vi "MoveOneStep.vi"(8 "error in (no error)":errorcluster, 11 "SnakeBodyUnit in":refnum<class "SnakeBodyCell.lvclass">) -> (0 "error out":errorcluster, 3 "SnakeBodyUnit out":refnum<class "SnakeBodyCell.lvclass">)   [LabVIEW 2018, in "SnakeBodyCell.lvclass"]
uses:
  SnakeBodyCell.lvclass
  SnakeBodyCell.lvclass/SnakeBodyCell.ctl
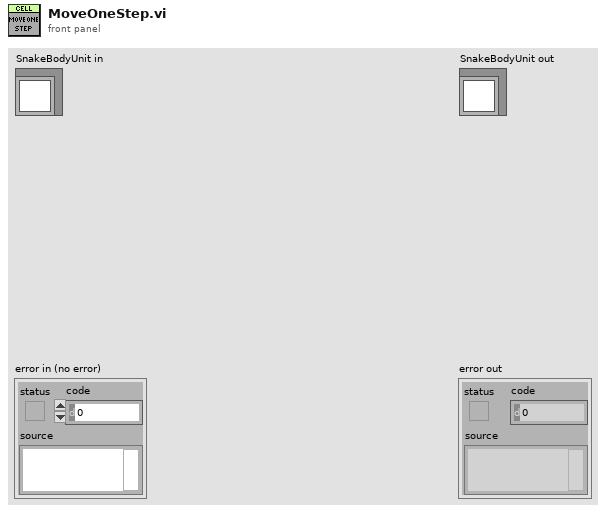
[diagram p1: front panel]
types:
  T1 = typedef "UnitDirection.ctl" = enum16{"North", "East", "South", "West"}
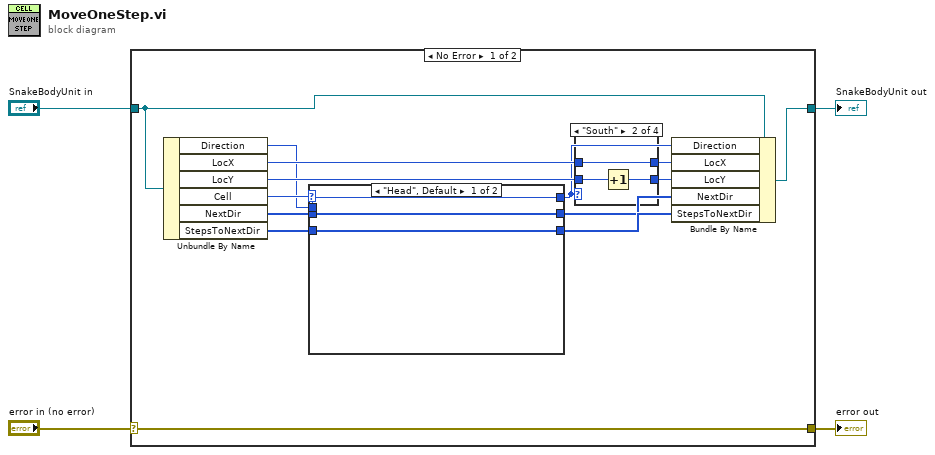
[diagram p0: block diagram]
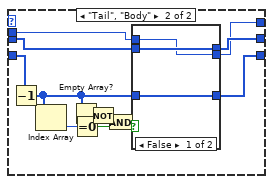
[diagram p2: hidden frame]
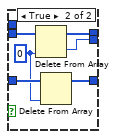
[diagram p3: hidden frame]
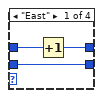
[diagram p4: hidden frame]
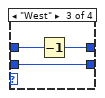
[diagram p5: hidden frame]
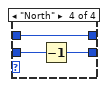
[diagram p6: hidden frame]
diagram:
  n1 = case shown="No Error" "error in (no error)" {
    selector: "error in (no error)" -> [w18 w56]
    tunnel: [w18 w56] -> w3
    tunnel: [w16 w55] -> w1
    tunnel: "SnakeBodyUnit in" -> [w17 w55]
    frame No Error {
      n2 = Unbundle By Name(w17) -> ("Direction"=w7:T1, "LocX"=w14:u16, "LocY"=w12:u16, "Cell"=w11:enum16{"Head", "Tail", "Body"}, "NextDir"=w9:T1[], "StepsToNextDir"=w10:u16[])
      n3 = case shown="\"Head\", Default" w11 {
        tunnel: w10 -> [w20 w33]
        tunnel: w9 -> [w19 w31]
        tunnel: [w20 w29] -> w8
        tunnel: [w21 w28] -> w5
        tunnel: w7 -> [w21 w26]
        tunnel: [w19 w30] -> w6
        frame "Head", Default {
        }
        frame "Tail", "Body" {
          n4 = Decrement(x=w33) -> (x-1=w23:u16[])
          n5 = Index Array(array=w23) -> (element=w32:u16)  [unwired: 1 in]
          n6 = Empty Array?(array=w23) -> (empty?=w24:bool)
          n7 = Equal To 0?(x=w32) -> (x = 0?=w27:bool)
          n8 = Not(x=w24) -> (.not. x?=w22:bool)
          n9 = And(x=w22, y=w27) -> (x .and. y?=w25:bool)
          n10 = case shown="False" w25 {
            tunnel: w23 -> [w35 w42]
            tunnel: w31 -> [w36 w41]
            tunnel: [w36 w40] -> w30
            tunnel: [w35 w39] -> w29
            tunnel: [w34 w37] -> w28
            tunnel: w26 -> [w34 _]
            frame False {
            }
            frame True {
              w38 = 0 ("index")
              n11 = Delete From Array(array=w41, index=w38) -> (deleted portion=w37:T1, array with subset deleted=w40:T1[])  [unwired: 1 in]
              n12 = Delete From Array(array=w42, index=w38) -> (array with subset deleted=w39:u16[])  [unwired: 1 in, 1 out]
            }
          }
        }
      }
      n13 = case shown="\"South\"" w5 {
        tunnel: [w43 w48 w49 w54] -> w15
        tunnel: w14 -> [w45 w48 w51 w54]
        tunnel: [w44 w46 w50 w52] -> w13
        tunnel: w12 -> [w44 w47 w50 w53]
        frame "East" {
          n14 = Increment(x=w45) -> (x+1=w43:u16)
        }
        frame "South" {
          n15 = Increment(x=w47) -> (x+1=w46:u16)
        }
        frame "West" {
          n16 = Decrement(x=w51) -> (x-1=w49:u16)
        }
        frame "North" {
          n17 = Decrement(x=w53) -> (x-1=w52:u16)
        }
      }
      n18 = Bundle By Name(cluster=w17, "Direction"=w5, "LocX"=w15, "LocY"=w13, "NextDir"=w6, "StepsToNextDir"=w8) -> (w16:refnum<class "SnakeBodyCell.lvclass">)
    }
    frame Error {
    }
  }
  "error out" <- w3
  "SnakeBodyUnit out" <- w1
